vi "SQLFreeHandle.vi"(4 "error in (no error)":errorcluster, 6 "HandleType":T1(ring)=enum."SQL_HANDLE_ENV", 7 "InputHandle":i32) -> (0 "error out":errorcluster)   [LabVIEW 2011]
doc: "Libere la mémoire occupée par un lien"
uses:
  Odbc32.dll
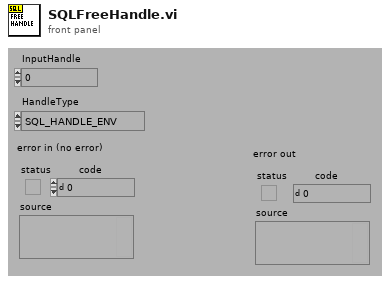
[diagram p1: front panel]
types:
  T1 = enum16{"NOPE", "SQL_HANDLE_ENV", "SQL_HANDLE_DBC", "SQL_HANDLE_STMT", "SQL_HANDLE_DESC"}
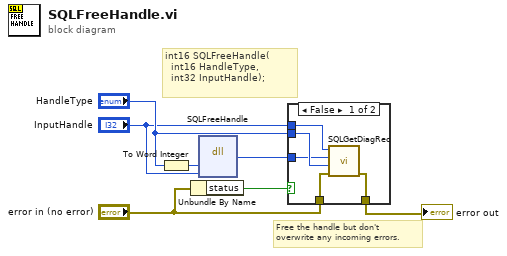
[diagram p0: block diagram]
diagram:
  # "Free the handle but don't\noverwrite any incoming errors."
  # "int16 SQLFreeHandle(\n  int16 HandleType, \n  int32 InputHandle);"
  n1 = To Word Integer(number="HandleType") -> (16bit integer=w4:i16)
  n2 = Unbundle By Name("error in (no error)") -> ("status"=w1:bool)
  n3 = dll-call lib="Odbc32.dll" fn="SQLFreeHandle"("HandleType"=w4, "InputHandle"="InputHandle") -> (w3:i16)  [unwired: 5 in, 2 out]
  n4 = case shown="False" w1 {
    tunnel: "HandleType" -> [w12 _]
    tunnel: "InputHandle" -> [w11 _]
    tunnel: [w10 w13] -> w5
    tunnel: w3 -> [w9 _]
    tunnel: "error in (no error)" -> [w8 w13]
    frame False {
      n5 = call "SQLGetDiagRec.vi"("error in (no error)"=w8, "HandleType"=w12, "Status (SQL_SUCCESS=0)"=w9, "Input Handle"=w11) -> ("error out"=w10:errorcluster)  [unwired: 3 out]
    }
    frame True {
    }
  }
  "error out" <- w5
